vi "Drop Field Encode.vi"(4 "Field":T1={"Name"="", "Number"=0, "Optional"=FALSE, "Repeated"=FALSE, "Type"={"Type"=enum."double", "Subtype"=""}, "Key Type"={"Type"=enum."double", "Subtype"=""}, "Value Type"={"Type"=enum."double", "Subtype"=""}}, 6 "Message Name":string, 7 "Value Terminal":refnum<vi>, 8 "error in (no error)":errorcluster, 9 "BD":refnum<vi>, 10 "Prev Term":refnum<vi>, 11 "LV-Protoc in":refnum<class "LV-Protoc.lvclass">) -> (0 "error out":errorcluster, 2 "Output Term":refnum<vi>, 3 "LV-Protoc out":refnum<class "LV-Protoc.lvclass">)   [LabVIEW 2020, in "LV-Protoc.lvlib" / "LV-Protoc.lvclass"]
uses:
  LV-Protoc.lvclass
  LV-Proto/Field.ctl
  LV-Proto/Type.ctl
  LV-Proto/Proto Type.ctl
  <vilib>/Utility/miscctls.llb/LVPointTypeDef.ctl
  Encode Terminal.ctl
  Flatten Terminal.ctl
  LV-Proto/LV-Proto.lvlib
  LV-Protoc.lvlib
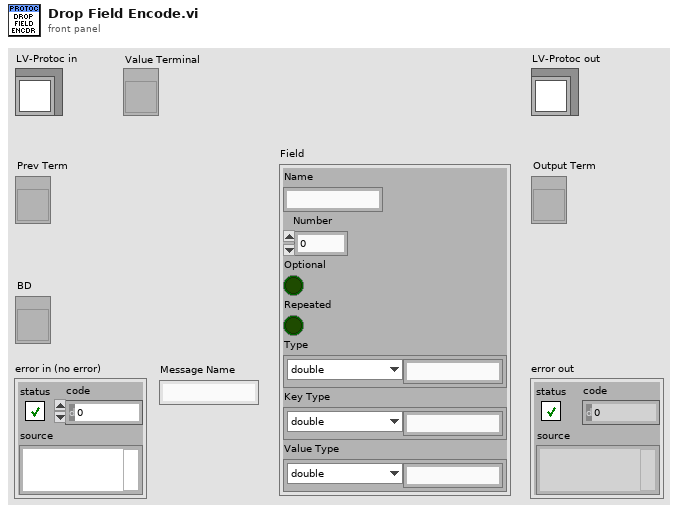
[diagram p1: front panel]
types:
  T1 = typedef "LV-Proto.lvlib/Field.ctl" = cluster{"Name":string, "Number":u32, "Optional":bool, "Repeated":bool, "Type":T2, "Key Type":T2, "Value Type":T2}
  T2 = typedef "LV-Proto.lvlib/Type.ctl" = cluster{"Type":T3, "Subtype":string}
  T3 = typedef "LV-Proto.lvlib/Proto Type.ctl" = enum16{"UNKNOWN", "double", "float", "int32", "int64", "uint32", "uint64", "sint32", "sint64", "fixed32", "fixed64", "sfixed32", "sfixed64", "bool", "string", "bytes", "enum", "map", "message"}
  T4 = typedef "LV-Protoc.lvlib/Encode Terminal.ctl" = enum16{"NA 0", "NA 1", "NA 2", "Buffer", "NA 4", "NA 5", "NA 6", "Field Number", "NA 8", "NA 9", "Value", "Buffer In"}
  T5 = typedef "LVPointTypeDef.ctl" = cluster{"Horizontal":i16, "Vertical":i16}
  T6 = typedef "LV-Protoc.lvlib/Flatten Terminal.ctl" = enum16{"error out", "NA 1", "Buffer", "NA 3", "NA 4", "NA 5", "NA 6", "NA 7", "error in", "Data", "NA 10", "NA 11"}
  T7 = typedef "LV-Protoc.lvlib/Enumeration Paths.ctl" = cluster{"Name":string, "Library":path, "Typedef":path, "Encode":path, "Encode packed":path, "Decode":path, "Decode packed":path, "Enum Value":path, "Enum from Value":path}
  T8 = typedef "LV-Protoc.lvlib/Message Paths.ctl" = cluster{"Name":string, "Library":path, "Data Typedef":path, "MessageName VI":path, "Flatten VI":path, "Unflatten VI":path, "Flatten repeated VI":path, "Decode VI":path}
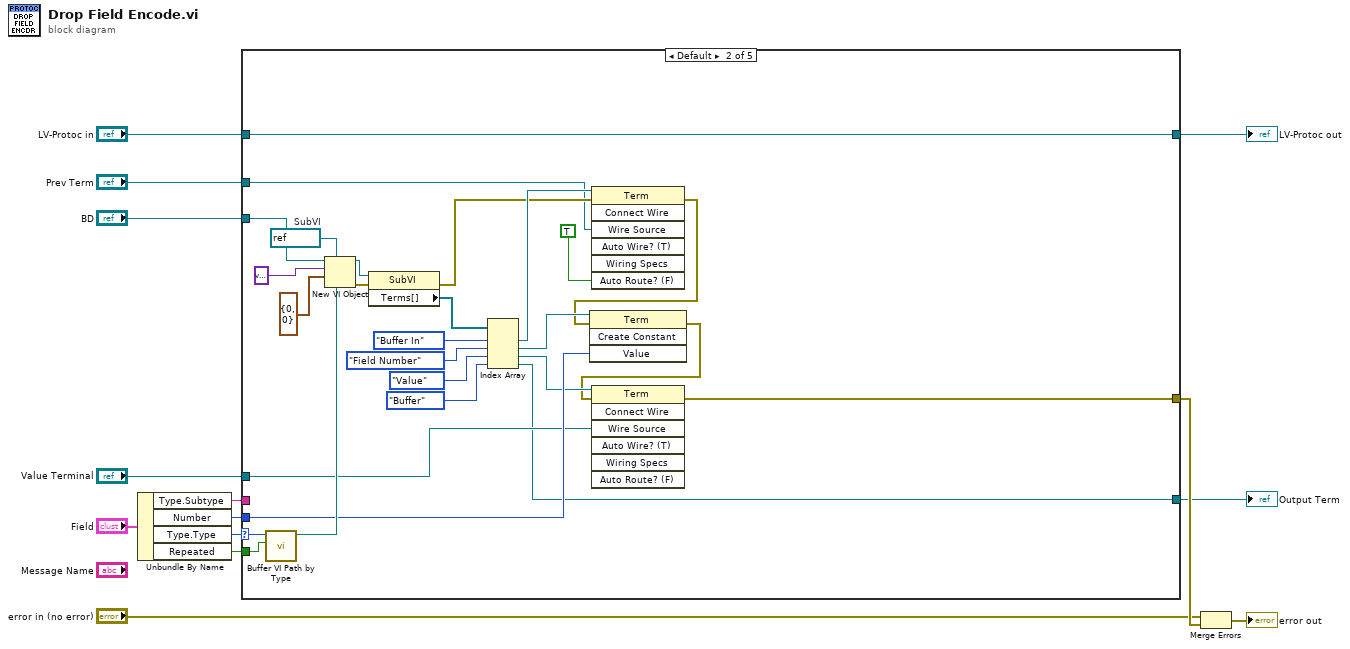
[diagram p0: block diagram]
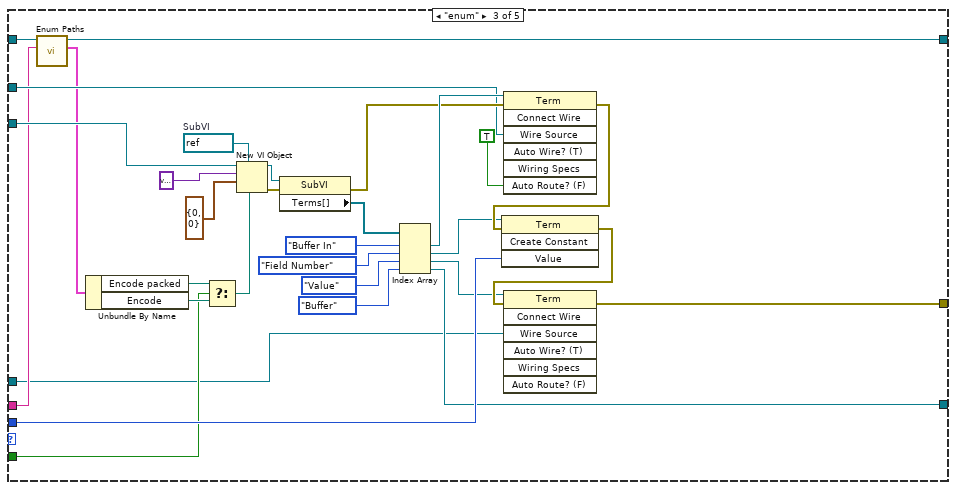
[diagram p3: hidden frame]
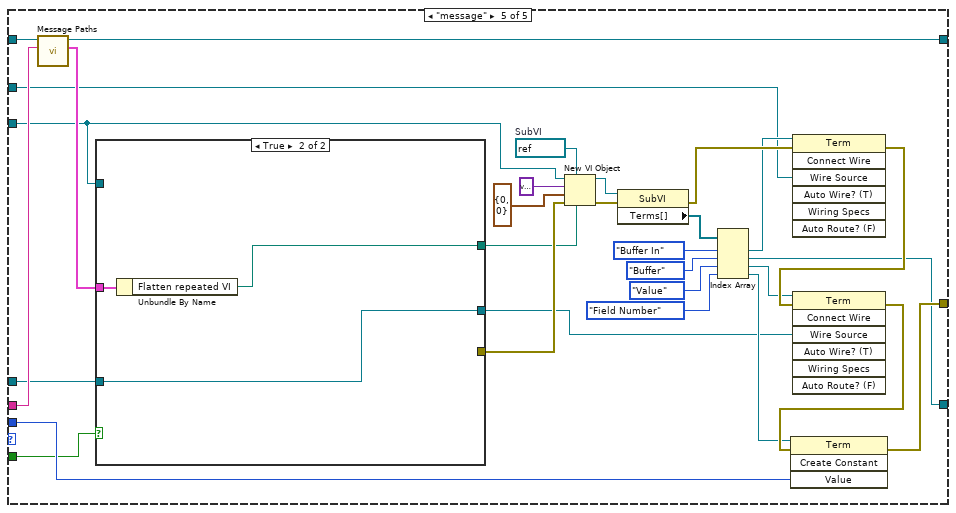
[diagram p5: hidden frame]
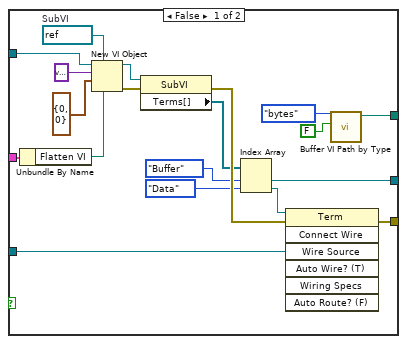
[diagram p6: hidden frame]
diagram:
  n1 = Unbundle By Name("Field") -> ("Type.Subtype"=w1:string, "Number"=w10:u32, "Type.Type"=w11:T3, "Repeated"=w2:bool)
  n2 = case shown="Default" w11 {
    selector: w11 -> [_ w43 _ _ _]
    tunnel: w10 -> [_ w24 w57 _ w84]
    tunnel: "BD" -> [_ w42 w53 _ w77]
    tunnel: [w16 w28 w50 w76 w101] -> w8
    tunnel: "LV-Protoc in" -> [w16 w28 w52 w76 w102]
    tunnel: "Prev Term" -> [w15 w26 w59 w75 w82]
    tunnel: "Value Terminal" -> [_ w21 w44 _ w98]
    tunnel: [w15 w19 w55 w75 w81] -> w4
    tunnel: [_ w18 w54 _ w103] -> w14
    tunnel: w2 -> [_ w17 w46 _ w78]
    tunnel: w1 -> [_ _ w51 _ w100]
    frame "UNKNOWN" {
    }
    frame Default {
      w38 = refnum<vi> refnum  # SubVI
      n3 = call "Buffer VI Path by Type.vi"("Repeated"=w17, "Proto Type"=w43) -> ("Encode"=w41:path)  [unwired: 8 in, 1 out]
      n4 = New VI Object(vi object class=w38, owner refnum=w42, style=variant, position/next to=T5 {"Horizontal"=0, "Vertical"=0} ("location"), 6:w41) -> (object refnum=w36:refnum<vi>, 0:w37:errorcluster)  [unwired: 3 in]
      n5 = property class="SubVI"(reference=w36, error in=w37) -> (error out=w27:errorcluster, "Terms[]"=w35:refnum<vi>[])  [unwired: 1 out]
      n6 = Index Array(array=w35, index #1=Encode_Terminal."Buffer In" ("Encode Terminal"), index #2=Encode_Terminal."Field Number" ("Encode Terminal"), index #3=Encode_Terminal."Value" ("Encode Terminal"), index #4=Encode_Terminal."Buffer" ("Encode Terminal")) -> (element #1=w30:refnum<vi>, element #2=w25:refnum<vi>, element #3=w22:refnum<vi>, element #4=w19:refnum<vi>)
      n7 = invoke class="Term" method="Connect Wire"(reference=w30, error in=w27, "Wire Source"=w26, "Auto Route? (F)"=TRUE) -> (error out=w23:errorcluster)  [unwired: 3 in, 6 out]
      n8 = invoke class="Term" method="Create Constant"(reference=w25, error in=w23, "Value"=w24) -> (error out=w20:errorcluster)  [unwired: 1 in, 3 out]
      n9 = invoke class="Term" method="Connect Wire"(reference=w22, error in=w20, "Wire Source"=w21) -> (error out=w18:errorcluster)  [unwired: 4 in, 6 out]
    }
    frame "enum" {
      w70 = refnum<vi> refnum  # SubVI
      n10 = call "Enum Paths.vi"("Enum Type Name"=w51, "LV-Protoc in"=w52) -> ("Enum Paths"=w49:T7, "LV-Protoc out"=w50:refnum<class "LV-Protoc.lvclass">)  [unwired: 7 in, 1 out]
      n11 = Unbundle By Name(w49) -> ("Encode packed"=w48:path, "Encode"=w47:path)
      n12 = Select(t=w48, s=w46, f=w47) -> (s? t:f=w45:path)
      n13 = New VI Object(vi object class=w70, owner refnum=w53, style=variant, position/next to=T5 {"Horizontal"=0, "Vertical"=0} ("location"), 6:w45) -> (object refnum=w68:refnum<vi>, 0:w69:errorcluster)  [unwired: 3 in]
      n14 = property class="SubVI"(reference=w68, error in=w69) -> (error out=w60:errorcluster, "Terms[]"=w67:refnum<vi>[])  [unwired: 1 out]
      n15 = Index Array(array=w67, index #1=Encode_Terminal."Buffer In" ("Encode Terminal"), index #2=Encode_Terminal."Field Number" ("Encode Terminal"), index #3=Encode_Terminal."Value" ("Encode Terminal"), index #4=Encode_Terminal."Buffer" ("Encode Terminal")) -> (element #1=w62:refnum<vi>, element #2=w58:refnum<vi>, element #3=w56:refnum<vi>, element #4=w55:refnum<vi>)
      n16 = invoke class="Term" method="Connect Wire"(reference=w62, error in=w60, "Wire Source"=w59, "Auto Route? (F)"=TRUE) -> (error out=w74:errorcluster)  [unwired: 3 in, 6 out]
      n17 = invoke class="Term" method="Create Constant"(reference=w58, error in=w74, "Value"=w57) -> (error out=w73:errorcluster)  [unwired: 1 in, 3 out]
      n18 = invoke class="Term" method="Connect Wire"(reference=w56, error in=w73, "Wire Source"=w44) -> (error out=w54:errorcluster)  [unwired: 4 in, 6 out]
    }
    frame "map" {
    }
    frame "message" {
      w97 = refnum<vi> refnum  # SubVI
      n19 = call "Message Paths.vi"("Message Type Name"=w100, "LV-Protoc in"=w102) -> ("Message Paths"=w99:T8, "LV-Protoc out"=w101:refnum<class "LV-Protoc.lvclass">)  [unwired: 7 in, 1 out]
      n20 = case shown="True" w78 {
        tunnel: w99 -> [w124 w128]
        tunnel: w98 -> [w113 w126]
        tunnel: w77 -> [w110 _]
        tunnel: [w109 _] -> w94
        tunnel: [w108 w127] -> w93
        tunnel: [w107 w126] -> w79
        frame False {
          w120 = refnum<vi> refnum  # SubVI
          n21 = Unbundle By Name(w124) -> ("Flatten VI"=w123:path)
          n22 = New VI Object(vi object class=w120, owner refnum=w110, style=variant, position/next to=T5 {"Horizontal"=0, "Vertical"=0} ("location"), 6:w123) -> (object refnum=w118:refnum<vi>, 0:w119:errorcluster)  [unwired: 3 in]
          n23 = property class="SubVI"(reference=w118, error in=w119) -> (error out=w125:errorcluster, "Terms[]"=w117:refnum<vi>[])  [unwired: 1 out]
          n24 = Index Array(array=w117, index #1=Flatten_Terminal."Buffer" ("Flatten Terminal"), index #2=Flatten_Terminal."Data" ("Flatten Terminal")) -> (element #1=w107:refnum<vi>, element #2=w114:refnum<vi>)
          n25 = invoke class="Term" method="Connect Wire"(reference=w114, error in=w125, "Wire Source"=w113) -> (error out=w109:errorcluster)  [unwired: 4 in, 6 out]
          n26 = call "Buffer VI Path by Type.vi"("Repeated"=FALSE ("Packed Repeated"), "Proto Type"=Proto_Type."bytes") -> ("Encode"=w108:path)  [unwired: 8 in, 1 out]
        }
        frame True {
          n27 = Unbundle By Name(w128) -> ("Flatten repeated VI"=w127:path)
        }
      }
      n28 = New VI Object(vi object class=w97, owner refnum=w77, style=variant, position/next to=T5 {"Horizontal"=0, "Vertical"=0} ("location"), 6:w93, 8:w94) -> (object refnum=w90:refnum<vi>, 0:w91:errorcluster)  [unwired: 2 in]
      n29 = property class="SubVI"(reference=w90, error in=w91) -> (error out=w106:errorcluster, "Terms[]"=w92:refnum<vi>[])  [unwired: 1 out]
      n30 = Index Array(array=w92, index #1=Encode_Terminal."Buffer In" ("Encode Terminal"), index #2=Encode_Terminal."Buffer" ("Encode Terminal"), index #3=Encode_Terminal."Value" ("Encode Terminal"), index #4=Encode_Terminal."Field Number" ("Encode Terminal")) -> (element #1=w83:refnum<vi>, element #2=w81:refnum<vi>, element #3=w80:refnum<vi>, element #4=w85:refnum<vi>)
      n31 = invoke class="Term" method="Connect Wire"(reference=w83, error in=w106, "Wire Source"=w82) -> (error out=w105:errorcluster)  [unwired: 4 in, 6 out]
      n32 = invoke class="Term" method="Connect Wire"(reference=w80, error in=w105, "Wire Source"=w79) -> (error out=w104:errorcluster)  [unwired: 4 in, 6 out]
      n33 = invoke class="Term" method="Create Constant"(reference=w85, error in=w104, "Value"=w84) -> (error out=w103:errorcluster)  [unwired: 1 in, 3 out]
    }
  }
  "LV-Protoc out" <- w8
  "Output Term" <- w4
  n34 = Merge Errors("error in (no error)", w14) -> (→"error out":errorcluster)
